vi "Get_Graph_Data.vi"(0 "Total_Data":T1[](array[typedef])) -> (4 "Array":dbl[][](array[numeric]))   [LabVIEW 2021]
doc: "Used to get the graph data from the generated data."
uses:
  Controls/Generated_data.ctl
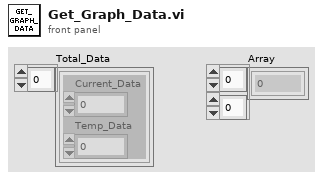
[diagram p1: front panel]
types:
  T1 = typedef "Generated_data.ctl" = cluster{"Current_Data":dbl, "Temp_Data":dbl}
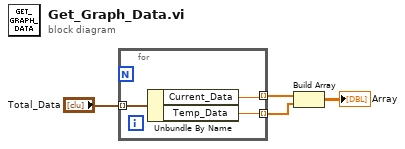
[diagram p0: block diagram]
diagram:
  n1 = for {
    tunnel: "Total_Data" -> [w7] mode=indexing
    tunnel: [w6] -> w1 mode=indexing
    tunnel: [w5] -> w2 mode=indexing
    n2 = Unbundle By Name(w7) -> ("Current_Data"=w6:dbl, "Temp_Data"=w5:dbl)
  }
  n3 = Build Array(w1, w2) -> (→"Array":dbl[][])
